vi "ADO Connection Open.vi"(8 "error in (no error)":errorcluster, 10 "ConnectionString":string, 11 "ADODB._Connection In":refnum<k7>) -> (0 "error out":errorcluster, 3 "ADODB._Connection Out":refnum<k7>)   [LabVIEW 2012]
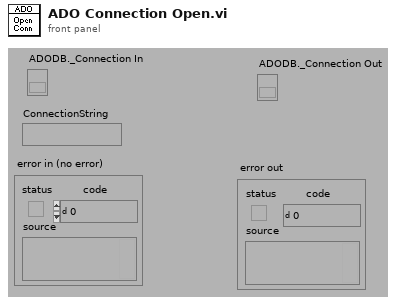
[diagram p1: front panel]
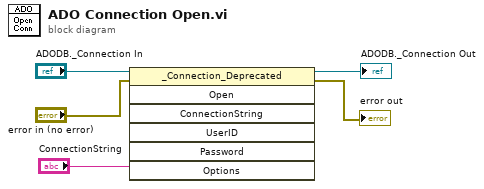
[diagram p0: block diagram]
diagram:
  n1 = invoke class="_Connection_Deprecated" method="Open"(reference="ADODB._Connection In", error in="error in (no error)", "ConnectionString"="ConnectionString") -> (reference out=→"ADODB._Connection Out":refnum<k7>, error out=→"error out":errorcluster)  [unwired: 4 in, 5 out]
